vi "Project_oldsteptext.vi"() -> ()   [LabVIEW 2023]
uses:
  <vilib>/Utility/file.llb/Read Delimited Spreadsheet (string).vi
  <instrlib>/Agilent N934X Series/Public/Configure/Measurement/Configure Measurement (Reflection Measurement).vi
  <instrlib>/Agilent N934X Series/Public/Configure/Measurement/Configure Measurement (Reflection Measurement - DTF).vi
  <instrlib>/Agilent N934X Series/Public/Configure/Configure Frequency (Reflection Measurement - Start Stop).vi
  <vilib>/Utility/file.llb/Write Delimited Spreadsheet (string).vi
  <instrlib>/Agilent N934X Series/Agilent N934X Series.lvlib
panel:
  in  "disabled?":bool
  in  "STOP":bool
  in  "Tab Control":enum32{"VSWR and Distance to Fault Test"}(tab)
  in  "Length of cable under test (ft)":dbl=5.0
  in  "Cable test":T1(ring)
  in  "VISA resource name":refnum<visa-resource-name>
  out "?":string
  out "Step:":i32
  out "Section:":string
  in  "Next step":bool
  out "Peak VSWR":dbl
  out "Peak frequency (MHz)":dbl
  out "Distance to fault (ft)":dbl
  # "(step image will go here)"
  # "Configuration"
  # "Results"
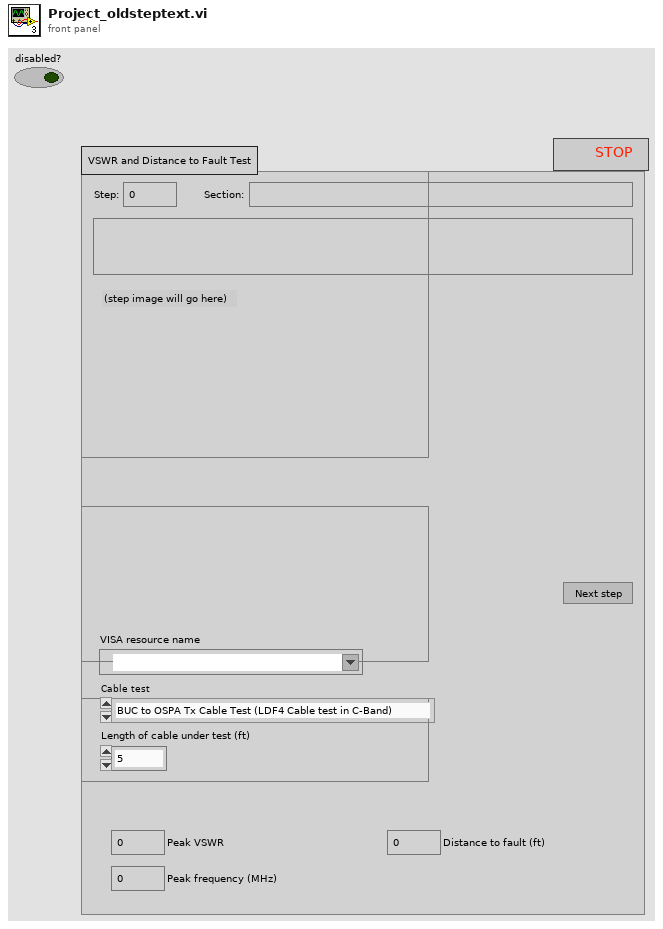
[diagram p1: front panel]
types:
  T1 = enum16{"BUC to OSPA Tx Cable Test (LDF4 Cable test in C-Band)", "BUC to OSPA Rx Cable Test (LDF4 Cable test in L-Band)", "Modem to BUC Tx Cable Test (LDF2 Cable test in L-Band)", "Modem to BUC Rx Cable Test (LDF2 Cable test in L-Band)"}
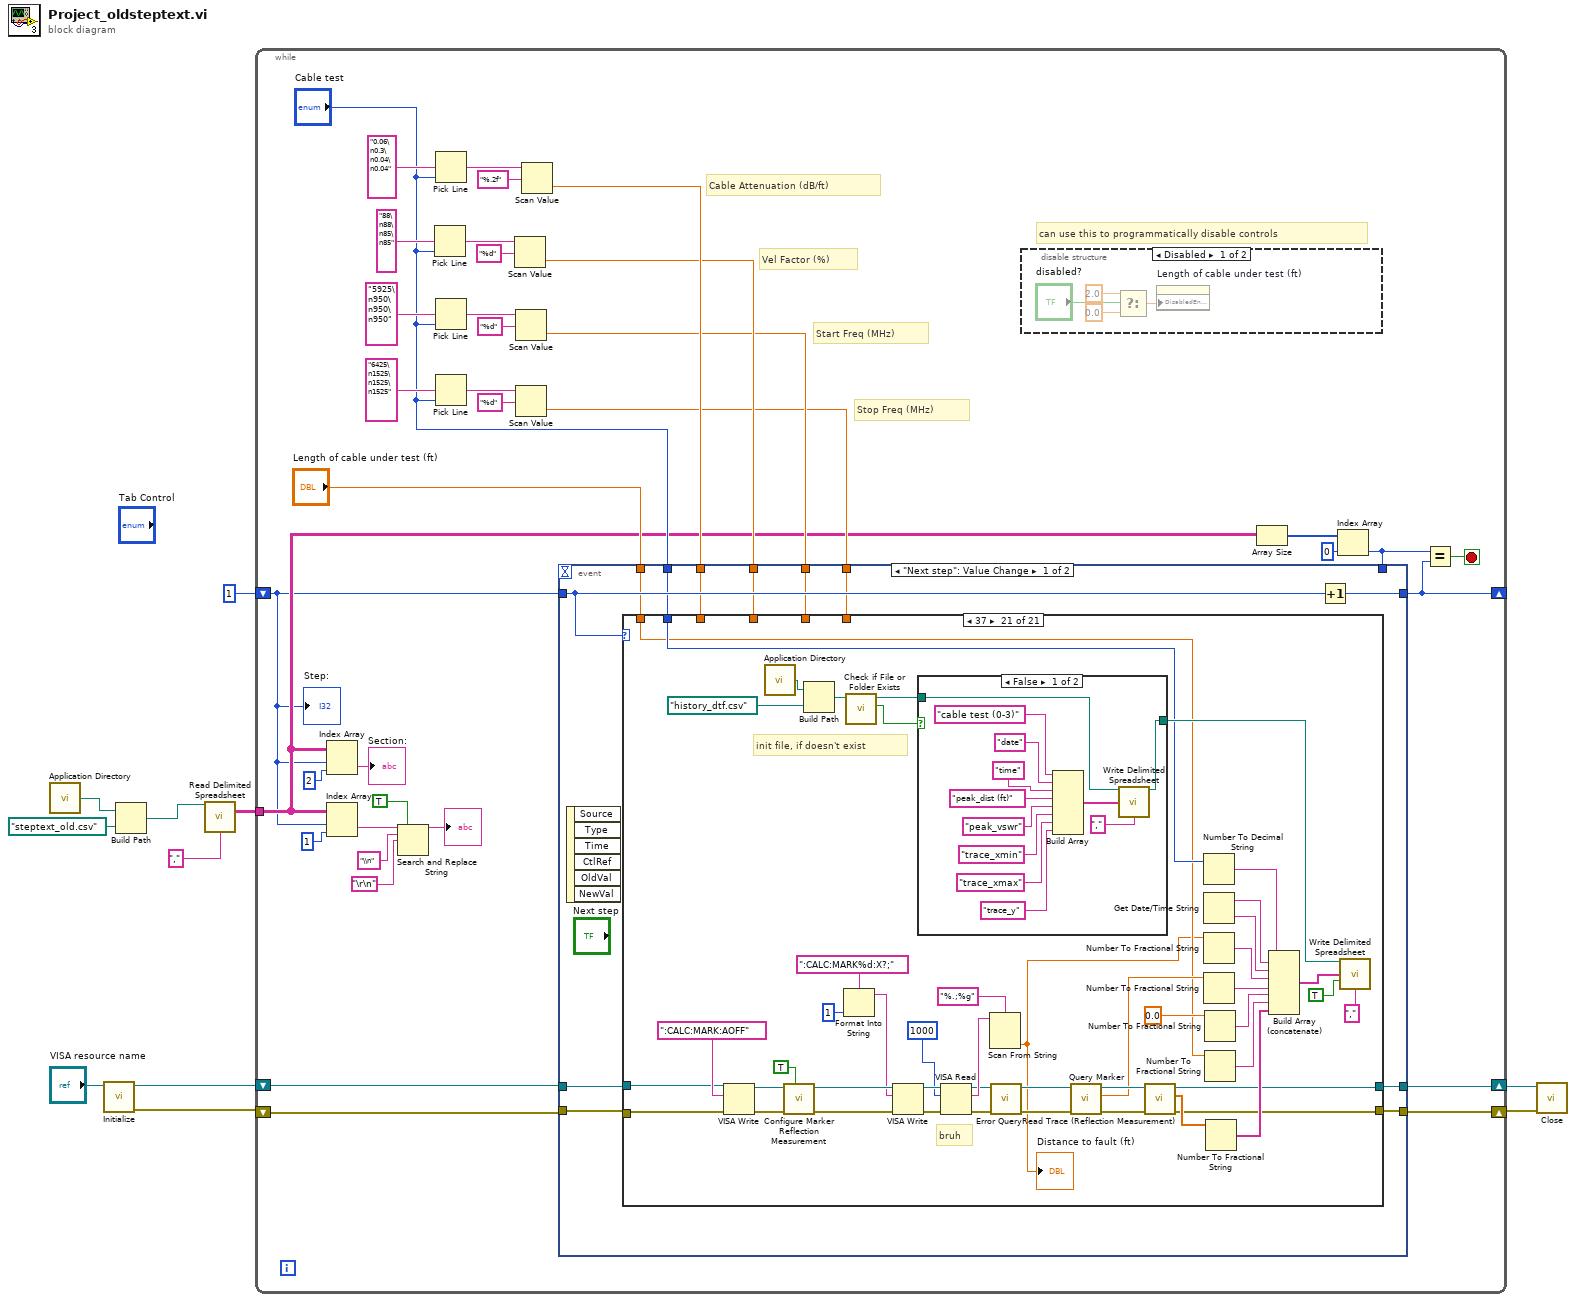
[diagram p0: block diagram]
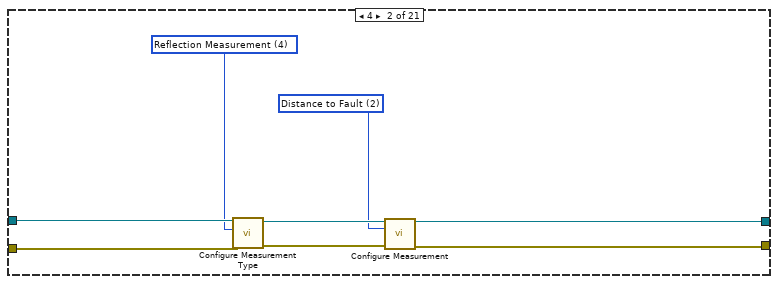
[diagram p4: hidden frame]
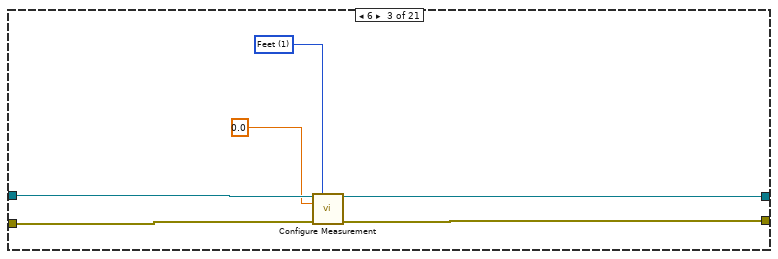
[diagram p5: hidden frame]
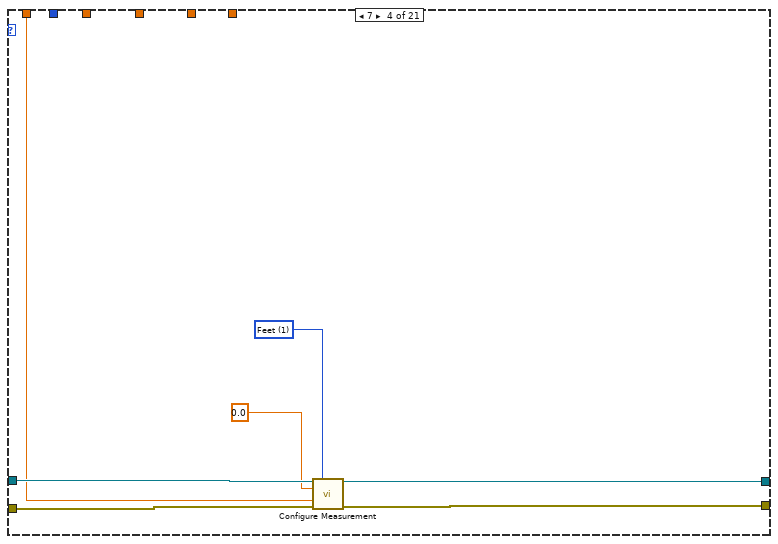
[diagram p6: hidden frame]
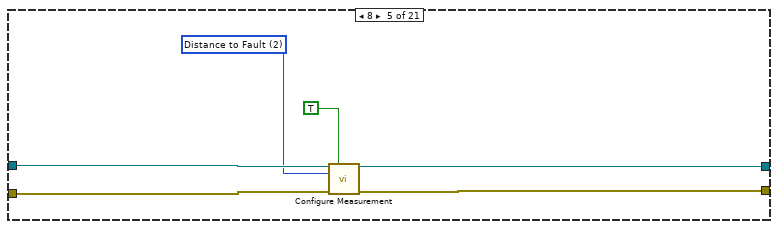
[diagram p7: hidden frame]
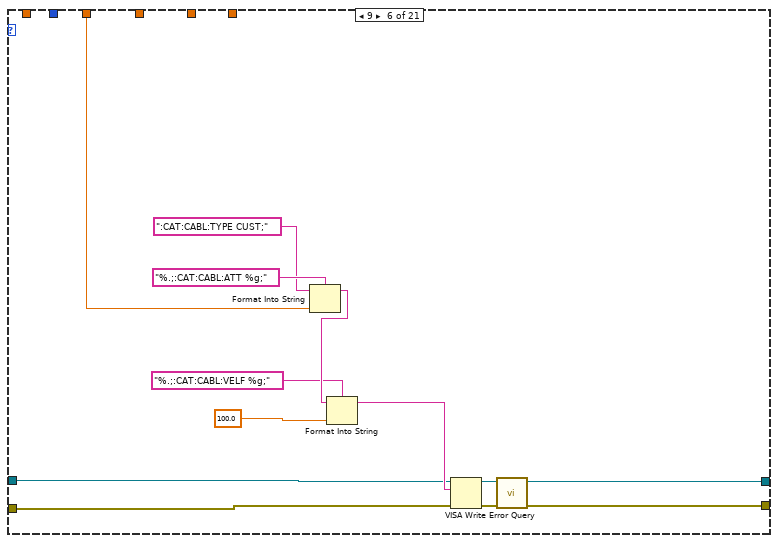
[diagram p8: hidden frame]
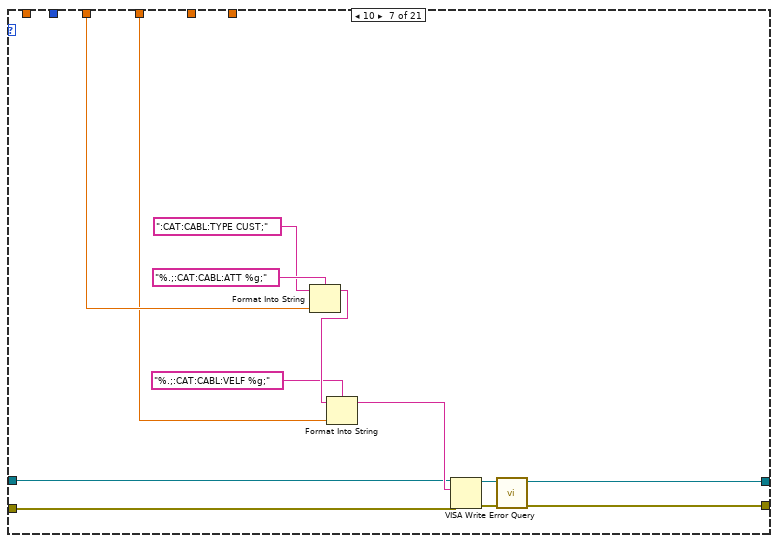
[diagram p9: hidden frame]
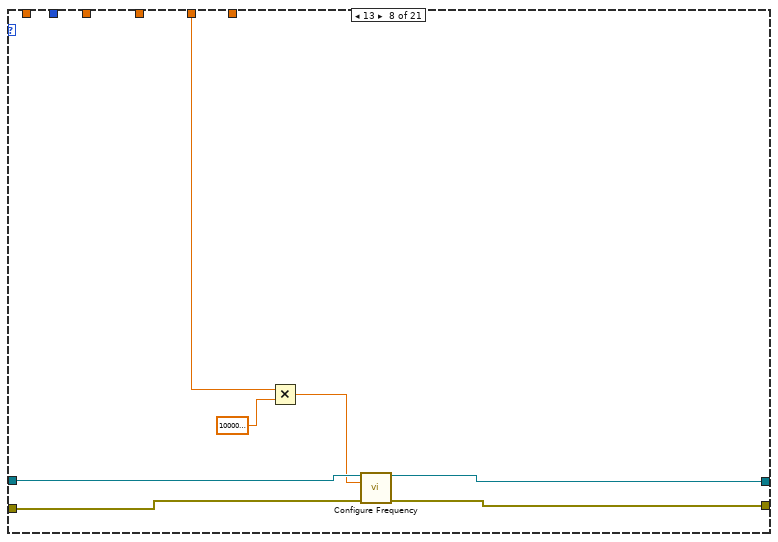
[diagram p10: hidden frame]
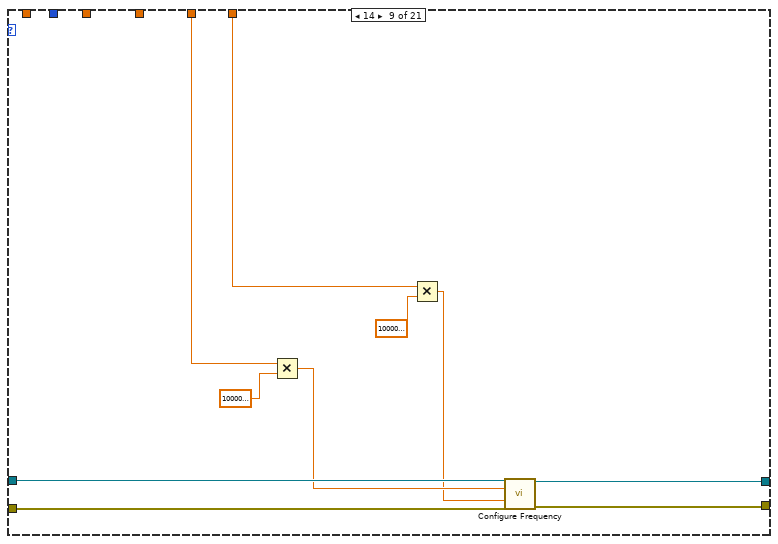
[diagram p11: hidden frame]
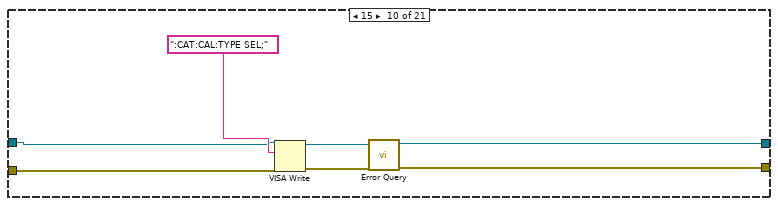
[diagram p12: hidden frame]
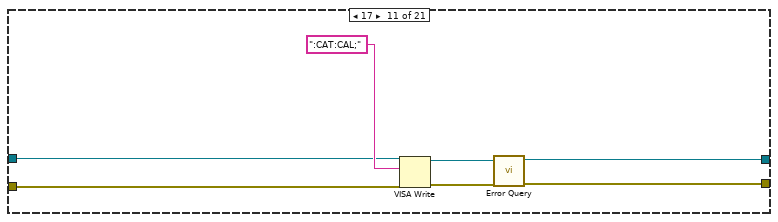
[diagram p13: hidden frame]
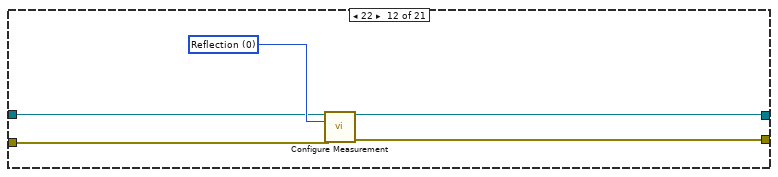
[diagram p14: hidden frame]
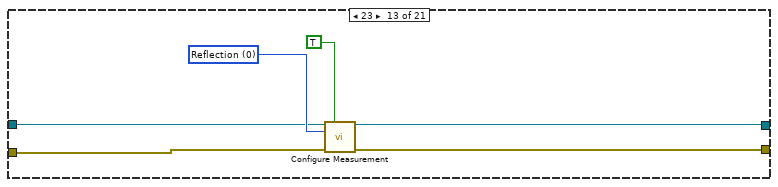
[diagram p15: hidden frame]
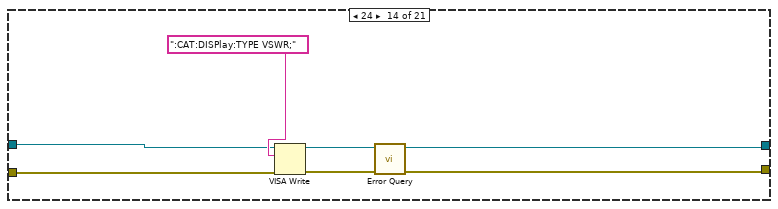
[diagram p16: hidden frame]
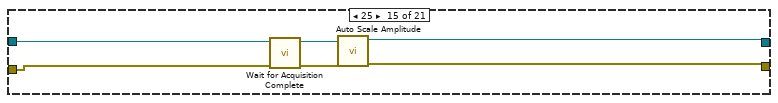
[diagram p17: hidden frame]
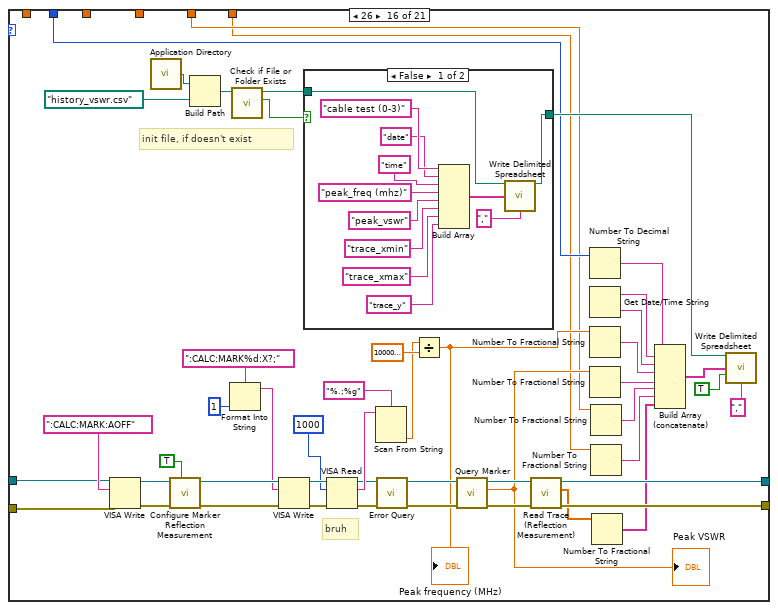
[diagram p18: hidden frame]
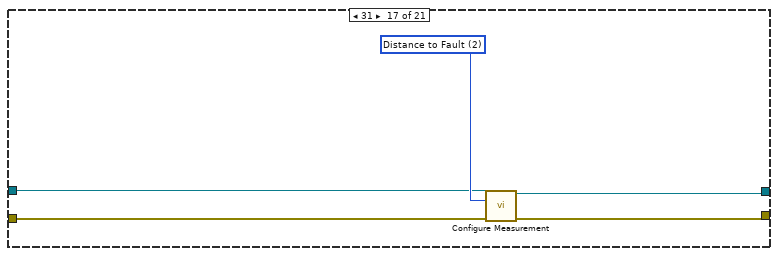
[diagram p20: hidden frame]
diagram:
  n1 = call <vilib>:"Application Directory.vi"() -> ("Application Directory"=w8:path)
  n2 = call <instrlib>:"Initialize.vi"("VISA resource name"="VISA resource name") -> ("error out"=w3:errorcluster, "VISA resource name out"=w4:refnum<visa-resource-name>)  [unwired: 9 in]
  n3 = Build Path(base path=w8, name or relative path=path "steptext_old.csv") -> (appended path=w6:path)
  n4 = call-poly <vilib>:"Read Delimited Spreadsheet.vi"("file path (dialog if empty)"=w6, "delimiter (\\t)"="," ("delimiter (\\t)")) -> ("all rows"=w9:string[][])  [unwired: 8 in, 5 out]
  n5 = while {
    shift-right: [w15] -> _
    shift-left: 1 -> [w12]
    tunnel: w9 -> [w18]
    shift-right: [w45] -> w2
    shift-left: w4 -> [w43]
    shift-right: [w44] -> w1
    shift-left: w3 -> [w42]
    stop <- w14 stop-if-true
    # "can use this to programmatically disable controls"
    # "Stop Freq (MHz)"
    # "Start Freq (MHz)"
    # "Vel Factor (%)"
    # "Cable Attenuation (dB/ft)"
    n6 = Index Array(array=w18, index (row)=w12, index (col)=2) -> (element=→"Section:":string)
    n7 = Index Array(array=w18, index (row)=w12, index (col)=1) -> (element=w22:string)
    n8 = Search and Replace String(replace all?=TRUE ("replace all? (F)"), input string=w22, search string="\\n", replace string="\r\n") -> (result string=→"?":string)  [unwired: 4 in, 3 out]
    n9 = Pick Line(multi-line string="88\n88\n85\n85", line index="Cable test") -> (output string=w35:string)  [unwired: 1 in]
    n10 = Pick Line(multi-line string="0.06\n0.3\n0.04\n0.04", line index="Cable test") -> (output string=w36:string)  [unwired: 1 in]
    n11 = Pick Line(multi-line string="5925\n950\n950\n950", line index="Cable test") -> (output string=w32:string)  [unwired: 1 in]
    n12 = Pick Line(multi-line string="6425\n1525\n1525\n1525", line index="Cable test") -> (output string=w30:string)  [unwired: 1 in]
    n13 = Scan Value(string=w35, format string="%d") -> (value=w27:dbl)  [unwired: 1 in, 1 out]
    n14 = Scan Value(string=w32, format string="%d") -> (value=w26:dbl)  [unwired: 1 in, 1 out]
    n15 = Scan Value(string=w30, format string="%d") -> (value=w25:dbl)  [unwired: 1 in, 1 out]
    n16 = Scan Value(string=w36, format string="%.2f") -> (value=w28:dbl)  [unwired: 1 in, 1 out]
    n17 = disable-structure shown="Disabled" {
      frame Disabled {
        n18 = Select(t=2.0, s="disabled?", f=0.0) -> (s? t:f=w52:dbl)
        n19 = property on="Length of cable under test (ft)" class="DigNum (strict)"("DisabledEnum"=w52) -> ()  [unwired: 2 in, 2 out]
      }
      frame Enabled {
      }
    }
    n20 = Array Size(array=w18) -> (size(s)=w17:i32[])
    n21 = Index Array(array=w17, index=0) -> (element=w13:i32)
    n22 = event shown="[0] \"Next step\": Value Change" {
      selector: _ -> [_ _]
      dyn-events: _ -> [_ _]
      timeout: _ -> [_ _]
      tunnel: w12 -> [w59 _]
      tunnel: [w64 w323] -> w15
      tunnel: w43 -> [w63 w322]
      tunnel: w42 -> [w61 w321]
      tunnel: [w62 w322] -> w45
      tunnel: [w60 w321] -> w44
      tunnel: "Length of cable under test (ft)" -> [w58 _]
      tunnel: w28 -> [w57 _]
      tunnel: w27 -> [w56 _]
      tunnel: w26 -> [w55 _]
      tunnel: w25 -> [w54 _]
      tunnel: "Cable test" -> [w53 _]
      tunnel: w13 -> [_ w323]
      event "Next step": Value Change {
        n23 = event-data() -> ()  [unwired: 1 in, 6 out]
        n24 = case shown="37" w59 {
          tunnel: w63 -> [w66 w74 w80 w87 w93 w99 w112 w126 w136 w140 w147 w154 w160 w165 w170 w198 w238 w245 w251 w256 w267]
          tunnel: [w66 w68 w77 w84 w90 w96 w109 w123 w133 w137 w145 w152 w158 w163 w173 w184 w240 w243 w249 w260 w265] -> w62
          tunnel: w61 -> [w65 w73 w79 w86 w92 w98 w111 w125 w135 w139 w146 w153 w159 w164 w169 w197 w237 w244 w250 w255 w266]
          tunnel: [w65 w69 w78 w85 w91 w97 w110 w124 w134 w138 w144 w151 w157 w162 w174 w185 w239 w242 w248 w259 w264] -> w60
          tunnel: w58 -> [_ _ _ w81 _ _ _ _ _ _ _ _ _ _ _ _ _ _ _ _ w262]
          tunnel: w57 -> [_ _ _ _ _ w94 w108 _ _ _ _ _ _ _ _ _ _ _ _ _ _]
          tunnel: w56 -> [_ _ _ _ _ _ w107 _ _ _ _ _ _ _ _ _ _ _ _ _ _]
          tunnel: w55 -> [_ _ _ _ _ _ _ w122 w128 _ _ _ _ _ _ w176 _ _ _ _ _]
          tunnel: w54 -> [_ _ _ _ _ _ _ _ w127 _ _ _ _ _ _ w175 _ _ _ _ _]
          tunnel: w53 -> [_ _ _ _ _ _ _ _ _ _ _ _ _ _ _ w181 _ _ _ _ w268]
          frame Default {
          }
          frame 4 {
            w67 = 2 items=["Reflection", "One Port Insertion Loss", "Distance to Fault"] ("Measurement Type (0: Reflection)")
            w72 = 4 items=["Spectrum Analyzer", "Tracking Generator", "Power Meter", "Modulation Analyzer", "Reflection Measurement"] ("Measurement Type (0: Spectrum Analyzer)")
            n25 = call <instrlib>:"Configure Measurement Type.vi"("error in (no error)"=w73, "Measurement Type (0: Spectrum Analyzer)"=w72, "VISA resource name"=w74) -> ("error out"=w70:errorcluster, "VISA resource name out"=w71:refnum<visa-resource-name>)  [unwired: 7 in]
            n26 = call-poly <instrlib>:"Configure Measurement.vi"("VISA resource name"=w71, "Measurement Type (0: Reflection)"=w67, "error in (no error)"=w70) -> ("VISA resource name out"=w68:refnum<visa-resource-name>, "error out"=w69:errorcluster)  [unwired: 11 in]
          }
          frame 6 {
            w76 = 1 items=["Meter", "Feet"] ("Distance Unit (0: Meter)")
            n27 = call-poly <instrlib>:"Configure Measurement.vi"("VISA resource name"=w80, "Distance Unit (0: Meter)"=w76, "Distance Start (0.12 meters)"=0.0, "error in (no error)"=w79) -> ("VISA resource name out"=w77:refnum<visa-resource-name>, "error out"=w78:errorcluster)  [unwired: 10 in]
          }
          frame 7 {
            w83 = 1 items=["Meter", "Feet"] ("Distance Unit (0: Meter)")
            n28 = call-poly <instrlib>:"Configure Measurement.vi"("VISA resource name"=w87, "Distance Unit (0: Meter)"=w83, "Distance Start (0.12 meters)"=0.0, "Distance Stop (0.15 meter)"=w81, "error in (no error)"=w86) -> ("VISA resource name out"=w84:refnum<visa-resource-name>, "error out"=w85:errorcluster)  [unwired: 9 in]
          }
          frame 8 {
            w88 = 2 items=["Reflection", "One Port Insertion Loss", "Distance to Fault"] ("Measurement Type (0: Reflection)")
            n29 = call-poly <instrlib>:"Configure Measurement.vi"("VISA resource name"=w93, "Enable IIM (F: Disable)"=TRUE, "Measurement Type (0: Reflection)"=w88, "error in (no error)"=w92) -> ("VISA resource name out"=w90:refnum<visa-resource-name>, "error out"=w91:errorcluster)  [unwired: 10 in]
          }
          frame 9 {
            n30 = Format Into String(format string="%.;:CAT:CABL:ATT %g;", initial string=":CAT:CABL:TYPE CUST;" ("output string"), w94) -> (resulting string=w105:string)  [unwired: 1 in, 1 out]
            n31 = Format Into String(format string="%.;:CAT:CABL:VELF %g;", initial string=w105, 100.0 ("input 1")) -> (resulting string=w106:string)  [unwired: 1 in, 1 out]
            n32 = VISA Write(VISA resource name=w99, write buffer=w106, error in (no error)=w98) -> (VISA resource name out=w103:refnum<visa-resource-name>, error out=w104:errorcluster)  [unwired: 1 out]
            n33 = call <instrlib>:"Error Query.vi"("error in (no error)"=w104, "VISA resource name"=w103) -> ("error out"=w97:errorcluster, "VISA resource name out"=w96:refnum<visa-resource-name>)  [unwired: 6 in, 2 out]
          }
          frame 10 {
            n34 = Format Into String(format string="%.;:CAT:CABL:ATT %g;", initial string=":CAT:CABL:TYPE CUST;" ("output string"), w108) -> (resulting string=w118:string)  [unwired: 1 in, 1 out]
            n35 = Format Into String(format string="%.;:CAT:CABL:VELF %g;", initial string=w118, w107) -> (resulting string=w119:string)  [unwired: 1 in, 1 out]
            n36 = VISA Write(VISA resource name=w112, write buffer=w119, error in (no error)=w111) -> (VISA resource name out=w116:refnum<visa-resource-name>, error out=w117:errorcluster)  [unwired: 1 out]
            n37 = call <instrlib>:"Error Query.vi"("error in (no error)"=w117, "VISA resource name"=w116) -> ("error out"=w110:errorcluster, "VISA resource name out"=w109:refnum<visa-resource-name>)  [unwired: 6 in, 2 out]
          }
          frame 13 {
            n38 = Multiply(x=w122, y=1000000.0) -> (x*y=w120:dbl)
            n39 = call-poly <instrlib>:"Configure Frequency.vi"("VISA resource name"=w126, "Start Frequency (5E+6 Hz)"=w120, "error in (no error)"=w125) -> ("VISA resource name out"=w123:refnum<visa-resource-name>, "error out"=w124:errorcluster)  [unwired: 11 in]
          }
          frame 14 {
            n40 = Multiply(x=w128, y=1000000.0) -> (x*y=w130:dbl)
            n41 = Multiply(x=w127, y=1000000.0) -> (x*y=w129:dbl)
            n42 = call-poly <instrlib>:"Configure Frequency.vi"("VISA resource name"=w136, "Start Frequency (5E+6 Hz)"=w130, "Stop Frequency (5E+8 Hz)"=w129, "error in (no error)"=w135) -> ("VISA resource name out"=w133:refnum<visa-resource-name>, "error out"=w134:errorcluster)  [unwired: 10 in]
          }
          frame 15 {
            n43 = VISA Write(VISA resource name=w140, write buffer=":CAT:CAL:TYPE SEL;", error in (no error)=w139) -> (VISA resource name out=w143:refnum<visa-resource-name>, error out=w142:errorcluster)  [unwired: 1 out]
            n44 = call <instrlib>:"Error Query.vi"("error in (no error)"=w142, "VISA resource name"=w143) -> ("error out"=w138:errorcluster, "VISA resource name out"=w137:refnum<visa-resource-name>)  [unwired: 6 in, 2 out]
          }
          frame 17 {
            n45 = VISA Write(VISA resource name=w147, write buffer=":CAT:CAL;", error in (no error)=w146) -> (VISA resource name out=w150:refnum<visa-resource-name>, error out=w149:errorcluster)  [unwired: 1 out]
            n46 = call <instrlib>:"Error Query.vi"("error in (no error)"=w149, "VISA resource name"=w150) -> ("error out"=w144:errorcluster, "VISA resource name out"=w145:refnum<visa-resource-name>)  [unwired: 6 in, 2 out]
          }
          frame 22 {
            w155 = 0 items=["Reflection", "One Port Insertion Loss", "Distance to Fault"] ("Measurement Type (0: Reflection)")
            n47 = call-poly <instrlib>:"Configure Measurement.vi"("VISA resource name"=w154, "Measurement Type (0: Reflection)"=w155, "error in (no error)"=w153) -> ("VISA resource name out"=w152:refnum<visa-resource-name>, "error out"=w151:errorcluster)  [unwired: 11 in]
          }
          frame 23 {
            w161 = 0 items=["Reflection", "One Port Insertion Loss", "Distance to Fault"] ("Measurement Type (0: Reflection)")
            n48 = call-poly <instrlib>:"Configure Measurement.vi"("VISA resource name"=w160, "Enable IIM (F: Disable)"=TRUE, "Measurement Type (0: Reflection)"=w161, "error in (no error)"=w159) -> ("VISA resource name out"=w158:refnum<visa-resource-name>, "error out"=w157:errorcluster)  [unwired: 10 in]
          }
          frame 24 {
            n49 = VISA Write(VISA resource name=w165, write buffer=":CAT:DISPlay:TYPE VSWR;", error in (no error)=w164) -> (VISA resource name out=w167:refnum<visa-resource-name>, error out=w168:errorcluster)  [unwired: 1 out]
            n50 = call <instrlib>:"Error Query.vi"("error in (no error)"=w168, "VISA resource name"=w167) -> ("error out"=w162:errorcluster, "VISA resource name out"=w163:refnum<visa-resource-name>)  [unwired: 6 in, 2 out]
          }
          frame 25 {
            n51 = call <instrlib>:"Wait for Acquisition Complete.vi"("error in (no error)"=w169, "VISA resource name"=w170) -> ("error out"=w171:errorcluster, "VISA resource name out"=w172:refnum<visa-resource-name>)  [unwired: 8 in]
            n52 = call <instrlib>:"Auto Scale Amplitude.vi"("error in (no error)"=w171, "VISA resource name"=w172) -> ("error out"=w174:errorcluster, "VISA resource name out"=w173:refnum<visa-resource-name>)  [unwired: 8 in]
          }
          frame 26 {
            # "init file, if doesn't exist"
            # "bruh"
            n53 = VISA Write(VISA resource name=w198, write buffer=":CALC:MARK:AOFF", error in (no error)=w197) -> (VISA resource name out=w211:refnum<visa-resource-name>, error out=w212:errorcluster)  [unwired: 1 out]
            n54 = call <vilib>:"Application Directory.vi"() -> ("Application Directory"=w207:path)
            n55 = call <instrlib>:"Configure Marker Reflection Measurement.vi"("Enable Continuous Peak (F: Disable)"=TRUE, "error in (no error)"=w212, "VISA resource name"=w211) -> ("error out"=w219:errorcluster, "VISA resource name out"=w221:refnum<visa-resource-name>)  [unwired: 7 in]
            n56 = Build Path(base path=w207, name or relative path=path "history_vswr.csv") -> (appended path=w195:path)
            n57 = Format Into String(format string=":CALC:MARK%d:X?;", 1 ("input 1")) -> (resulting string=w213:string)  [unwired: 2 in, 1 out]
            n58 = call <vilib>:"Check if File or Folder Exists.vi"("path"=w195) -> ("file or folder exists?"=w192:bool, "dup path"=w194:path)  [unwired: 8 in, 1 out]
            n59 = VISA Write(VISA resource name=w221, write buffer=w213, error in (no error)=w219) -> (VISA resource name out=w214:refnum<visa-resource-name>, error out=w215:errorcluster)  [unwired: 1 out]
            n60 = case shown="False" w192 {
              tunnel: w194 -> [w224 w236]
              tunnel: [w225 w236] -> w193
              frame False {
                n61 = Build Array("cable test (0-3)" ("element"), "date" ("element"), "time" ("element"), "peak_freq (mhz)" ("element"), "peak_vswr" ("element"), "trace_xmin" ("element"), "trace_xmax" ("element"), "trace_y" ("element")) -> (w235:string[])
                n62 = call-poly <vilib>:"Write Delimited Spreadsheet.vi"("file path (dialog if empty)"=w224, "1D data"=w235, "delimiter (\\t)"="," ("delimiter (\\t)")) -> ("new file path (Not A Path if cancelled)"=w225:path)  [unwired: 11 in, 1 out]
              }
              frame True {
              }
            }
            n63 = VISA Read(VISA resource name=w214, byte count=u32 1000, error in (no error)=w215) -> (VISA resource name out=w216:refnum<visa-resource-name>, read buffer=w218:string, error out=w217:errorcluster)  [unwired: 1 out]
            n64 = Scan From String(format string="%.;%g", input string=w218) -> (output 1=w189:dbl)  [unwired: 3 in, 3 out]
            n65 = call <instrlib>:"Error Query.vi"("error in (no error)"=w217, "VISA resource name"=w216) -> ("error out"=w220:errorcluster, "VISA resource name out"=w222:refnum<visa-resource-name>)  [unwired: 6 in, 2 out]
            n66 = Divide(x=w189, y=1000000.0) -> (x/y=w188:dbl)
            "Peak frequency (MHz)" <- w188
            n67 = call <instrlib>:"Query Marker.vi"("error in (no error)"=w220, "VISA resource name"=w222) -> ("error out"=w186:errorcluster, "Y Value"=w179:dbl, "VISA resource name out"=w187:refnum<visa-resource-name>)  [unwired: 7 in]
            "Peak VSWR" <- w179
            n68 = call <instrlib>:"Read Trace (Reflection Measurement).vi"("error in (no error)"=w186, "VISA resource name"=w187) -> ("error out"=w185:errorcluster, "Trace Data"=w183:dbl[], "VISA resource name out"=w184:refnum<visa-resource-name>)  [unwired: 7 in]
            n69 = Number To Decimal String(number=w181) -> (decimal integer string=w182:string)  [unwired: 1 in]
            n70 = Get Date/Time String() -> (date string=w209:string, time string=w210:string)  [unwired: 3 in]
            n71 = Number To Fractional String(number=w188) -> (F-format string=w191:string)  [unwired: 3 in]
            n72 = Number To Fractional String(number=w179) -> (F-format string=w223:string)  [unwired: 3 in]
            n73 = Number To Fractional String(number=w176) -> (F-format string=w178:string)  [unwired: 3 in]
            n74 = Number To Fractional String(number=w175) -> (F-format string=w177:string)  [unwired: 3 in]
            n75 = Number To Fractional String(number=w183) -> (F-format string=w180:string[])  [unwired: 3 in]
            n76 = Build Array (concatenate)(w182, w209, w210, w191, w223, w178, w177, w180) -> (w208:string[])
            n77 = call-poly <vilib>:"Write Delimited Spreadsheet.vi"("file path (dialog if empty)"=w193, "1D data"=w208, "append to file? (new file:F)"=TRUE, "delimiter (\\t)"="," ("delimiter (\\t)")) -> ()  [unwired: 10 in, 2 out]
          }
          frame 31 {
            w241 = 2 items=["Reflection", "One Port Insertion Loss", "Distance to Fault"] ("Measurement Type (0: Reflection)")
            n78 = call-poly <instrlib>:"Configure Measurement.vi"("VISA resource name"=w238, "Measurement Type (0: Reflection)"=w241, "error in (no error)"=w237) -> ("VISA resource name out"=w240:refnum<visa-resource-name>, "error out"=w239:errorcluster)  [unwired: 11 in]
          }
          frame 32 {
            w247 = 2 items=["Reflection", "One Port Insertion Loss", "Distance to Fault"] ("Measurement Type (0: Reflection)")
            n79 = call-poly <instrlib>:"Configure Measurement.vi"("VISA resource name"=w245, "Enable IIM (F: Disable)"=FALSE, "Measurement Type (0: Reflection)"=w247, "error in (no error)"=w244) -> ("VISA resource name out"=w243:refnum<visa-resource-name>, "error out"=w242:errorcluster)  [unwired: 10 in]
          }
          frame 33 {
            n80 = VISA Write(VISA resource name=w251, write buffer=":CAT:DISPlay:TYPE VSWR;", error in (no error)=w250) -> (VISA resource name out=w253:refnum<visa-resource-name>, error out=w254:errorcluster)  [unwired: 1 out]
            n81 = call <instrlib>:"Error Query.vi"("error in (no error)"=w254, "VISA resource name"=w253) -> ("error out"=w248:errorcluster, "VISA resource name out"=w249:refnum<visa-resource-name>)  [unwired: 6 in, 2 out]
          }
          frame 34 {
            n82 = call <instrlib>:"Wait for Acquisition Complete.vi"("error in (no error)"=w255, "VISA resource name"=w256) -> ("error out"=w257:errorcluster, "VISA resource name out"=w258:refnum<visa-resource-name>)  [unwired: 8 in]
            n83 = call <instrlib>:"Auto Scale Amplitude.vi"("error in (no error)"=w257, "VISA resource name"=w258) -> ("error out"=w259:errorcluster, "VISA resource name out"=w260:refnum<visa-resource-name>)  [unwired: 8 in]
          }
          frame 37 {
            # "init file, if doesn't exist"
            # "bruh"
            n84 = VISA Write(VISA resource name=w267, write buffer=":CALC:MARK:AOFF", error in (no error)=w266) -> (VISA resource name out=w295:refnum<visa-resource-name>, error out=w296:errorcluster)  [unwired: 1 out]
            n85 = call <vilib>:"Application Directory.vi"() -> ("Application Directory"=w291:path)
            n86 = call <instrlib>:"Configure Marker Reflection Measurement.vi"("Enable Continuous Peak (F: Disable)"=TRUE, "error in (no error)"=w296, "VISA resource name"=w295) -> ("error out"=w303:errorcluster, "VISA resource name out"=w305:refnum<visa-resource-name>)  [unwired: 7 in]
            n87 = Build Path(base path=w291, name or relative path=path "history_dtf.csv") -> (appended path=w281:path)
            n88 = Format Into String(format string=":CALC:MARK%d:X?;", 1 ("input 1")) -> (resulting string=w297:string)  [unwired: 2 in, 1 out]
            n89 = call <vilib>:"Check if File or Folder Exists.vi"("path"=w281) -> ("file or folder exists?"=w278:bool, "dup path"=w280:path)  [unwired: 8 in, 1 out]
            n90 = VISA Write(VISA resource name=w305, write buffer=w297, error in (no error)=w303) -> (VISA resource name out=w298:refnum<visa-resource-name>, error out=w299:errorcluster)  [unwired: 1 out]
            n91 = case shown="False" w278 {
              tunnel: w280 -> [w308 w320]
              tunnel: [w309 w320] -> w279
              frame False {
                n92 = Build Array("cable test (0-3)" ("element"), "date" ("element"), "time" ("element"), "peak_dist (ft)" ("element"), "peak_vswr" ("element"), "trace_xmin" ("element"), "trace_xmax" ("element"), "trace_y" ("element")) -> (w319:string[])
                n93 = call-poly <vilib>:"Write Delimited Spreadsheet.vi"("file path (dialog if empty)"=w308, "1D data"=w319, "delimiter (\\t)"="," ("delimiter (\\t)")) -> ("new file path (Not A Path if cancelled)"=w309:path)  [unwired: 11 in, 1 out]
              }
              frame True {
              }
            }
            n94 = VISA Read(VISA resource name=w298, byte count=u32 1000, error in (no error)=w299) -> (VISA resource name out=w300:refnum<visa-resource-name>, read buffer=w302:string, error out=w301:errorcluster)  [unwired: 1 out]
            n95 = Scan From String(format string="%.;%g", input string=w302) -> (output 1=w261:dbl)  [unwired: 3 in, 3 out]
            "Distance to fault (ft)" <- w261
            n96 = call <instrlib>:"Error Query.vi"("error in (no error)"=w301, "VISA resource name"=w300) -> ("error out"=w304:errorcluster, "VISA resource name out"=w306:refnum<visa-resource-name>)  [unwired: 6 in, 2 out]
            n97 = call <instrlib>:"Query Marker.vi"("error in (no error)"=w304, "VISA resource name"=w306) -> ("error out"=w275:errorcluster, "Y Value"=w271:dbl, "VISA resource name out"=w276:refnum<visa-resource-name>)  [unwired: 7 in]
            n98 = call <instrlib>:"Read Trace (Reflection Measurement).vi"("error in (no error)"=w275, "VISA resource name"=w276) -> ("error out"=w264:errorcluster, "Trace Data"=w274:dbl[], "VISA resource name out"=w265:refnum<visa-resource-name>)  [unwired: 7 in]
            n99 = Number To Decimal String(number=w268) -> (decimal integer string=w273:string)  [unwired: 1 in]
            n100 = Get Date/Time String() -> (date string=w293:string, time string=w294:string)  [unwired: 3 in]
            n101 = Number To Fractional String(number=w261) -> (F-format string=w277:string)  [unwired: 3 in]
            n102 = Number To Fractional String(number=w271) -> (F-format string=w307:string)  [unwired: 3 in]
            n103 = Number To Fractional String(number=0.0) -> (F-format string=w270:string)  [unwired: 3 in]
            n104 = Number To Fractional String(number=w262) -> (F-format string=w269:string)  [unwired: 3 in]
            n105 = Number To Fractional String(number=w274) -> (F-format string=w272:string[])  [unwired: 3 in]
            n106 = Build Array (concatenate)(w273, w293, w294, w277, w307, w270, w269, w272) -> (w292:string[])
            n107 = call-poly <vilib>:"Write Delimited Spreadsheet.vi"("file path (dialog if empty)"=w279, "1D data"=w292, "append to file? (new file:F)"=TRUE, "delimiter (\\t)"="," ("delimiter (\\t)")) -> ()  [unwired: 10 in, 2 out]
          }
        }
        n108 = Increment(x=w59) -> (x+1=w64:i32)
      }
      event "STOP": Value Change {
        n109 = event-data() -> ()  [unwired: 1 in, 6 out]
      }
    }
    n110 = Equal?(x=w13, y=w15) -> (x = y?=w14:bool)
    "Step:" <- w12
  }
  n111 = call <instrlib>:"Close.vi"("error in (no error)"=w1, "VISA resource name"=w2) -> ()  [unwired: 9 in, 1 out]
